vi "FPGA_SPIWriteChipSelectActiveHigh.vi"(8 "error in (no error)":errorcluster, 10 "Chip Select Active High (F)":bool, 11 "SPI Bus":T1) -> (0 "error out":errorcluster)   [LabVIEW 2017]
uses:
  <vilib>/Rock Robotics/SystemInterfaces/spilib/spi_bus.ctl
  <vilib>/Utility/error.llb/Error Cluster From Error Code.vi
  <vilib>/rvi/errors/niLvFpgaAdjustHostInterfaceError.vi
  <vilib>/rvi/interface/nirviReadWriteControl/nirviReadWriteControl.xnode
  <vilib>/Rock Robotics/SystemInterfaces/System/FPGA_SystemFRC FPGA Ref.ctl
  <vilib>/rvi/interface/Simulation/niFpgaSimulationCallBeginRW.vi
  NiFpgaLv.dll
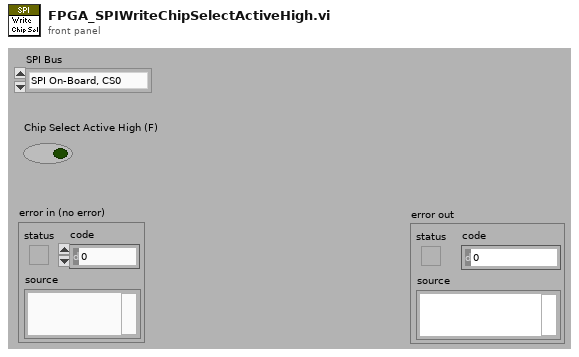
[diagram p1: front panel]
types:
  T1 = typedef "spi_bus.ctl" = enum16{"SPI On-Board, CS0", "SPI On-Board, CS1", "SPI On-Board, CS2", "SPI On-Board, CS3", "SPI MXP", "Invalid"}
  T2 = typedef "FPGA_SystemFRC FPGA Ref.ctl" = refnum<k20>
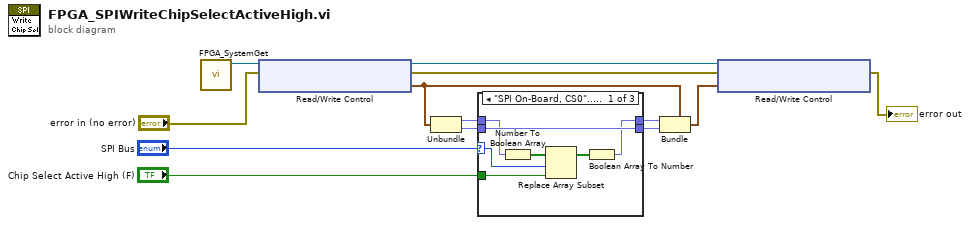
[diagram p0: block diagram]
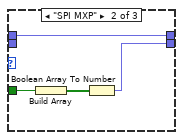
[diagram p2: hidden frame]
diagram:
  n1 = call <vilib>:"FPGA_SystemGet.vi"() -> ("FRC FPGA Ref"=w13:T2)  [unwired: 11 in]
  n2 = xnode "Read/Write Control"("FPGA VI Reference In"=w13, "error in"="error in (no error)") -> ("FPGA VI Reference Out"=w9:T2, "error out"=w8:errorcluster, "SPI.ChipSelectActiveHigh"=w11:cluster{"Hdr":fxp<+,4,4>, "MXP":fxp<+,1,1>})
  n3 = Unbundle(w11) -> ("Hdr"=w4:fxp<+,4,4>, "MXP"=w2:fxp<+,1,1>)
  n4 = case shown="\"SPI On-Board, CS0\"..\"SPI On-Board, CS3\"" "SPI Bus" {
    selector: "SPI Bus" -> [w15 _ _]
    tunnel: [w18 w24 w26] -> w5
    tunnel: w4 -> [w19 w24 w26]
    tunnel: [w20 w21 w25] -> w3
    tunnel: w2 -> [w20 _ w25]
    tunnel: "Chip Select Active High (F)" -> [w14 w23 _]
    frame "SPI On-Board, CS0".."SPI On-Board, CS3" {
      n5 = Number To Boolean Array(number=w19) -> (Boolean array=w17:bool[])
      n6 = Replace Array Subset(array=w17, new element=w14, index=w15) -> (w16:bool[])
      n7 = Boolean Array To Number(Boolean array=w16) -> (number=w18:fxp<+,4,4>)
    }
    frame "SPI MXP" {
      n8 = Build Array(w23) -> (w22:bool[])
      n9 = Boolean Array To Number(Boolean array=w22) -> (number=w21:fxp<+,1,1>)
    }
    frame "Invalid" {
      # "change nothing if invalid"
    }
  }
  n10 = Bundle(cluster=w11, "Hdr"=w5, "MXP"=w3) -> (w10:cluster{"Hdr":fxp<+,4,4>, "MXP":fxp<+,1,1>})
  n11 = xnode "Read/Write Control"("FPGA VI Reference In"=w9, "error in"=w8, "SPI.ChipSelectActiveHigh"=w10) -> ("error out"=→"error out":errorcluster)  [unwired: 1 out]
